vi "Run Test.vi"() -> ()   [LabVIEW 2026, in "Framework Engine.lvclass"]
uses:
  Framework Engine.lvclass
  Framework Engine.lvclass/Framework Engine.ctl
  Domain/Session/Session.lvclass
  Services/Readiness Service/Readines Service.lvclass
  Domain/Test Run Request/Test Run Request.lvclass
  Domain/User/User.lvclass
  Services/Execution Service/Execution Service.lvclass
panel:
  out "error out":errorcluster
  out "Test Run Request":refnum<class "Test Run Request.lvclass">
  in  "Package Version":string
  in  "Package ID":string
  in  "Entry Point":string
  in  "Sequence File Path":path
  in  "Station Name":string
  in  "error in (no error)":errorcluster
  out "Has Permission":bool
  out "Current User":refnum<class "User.lvclass">
  in  "Framework Engine in":refnum<class "Framework Engine.lvclass">
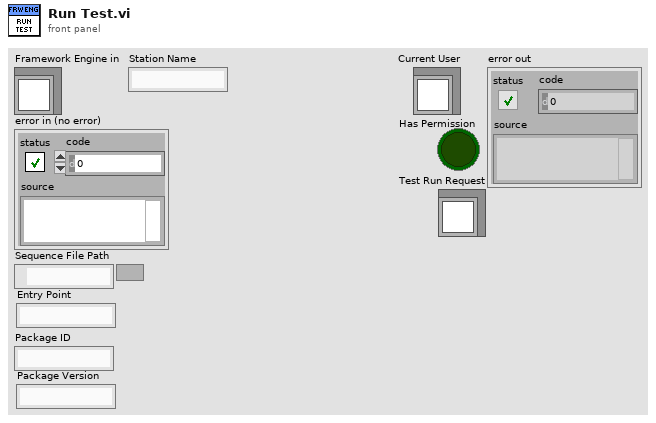
[diagram p1: front panel]
types:
  T1 = typedef "Role Enum.ctl" = enum16{"Operator", "Engineer", "Admin"}
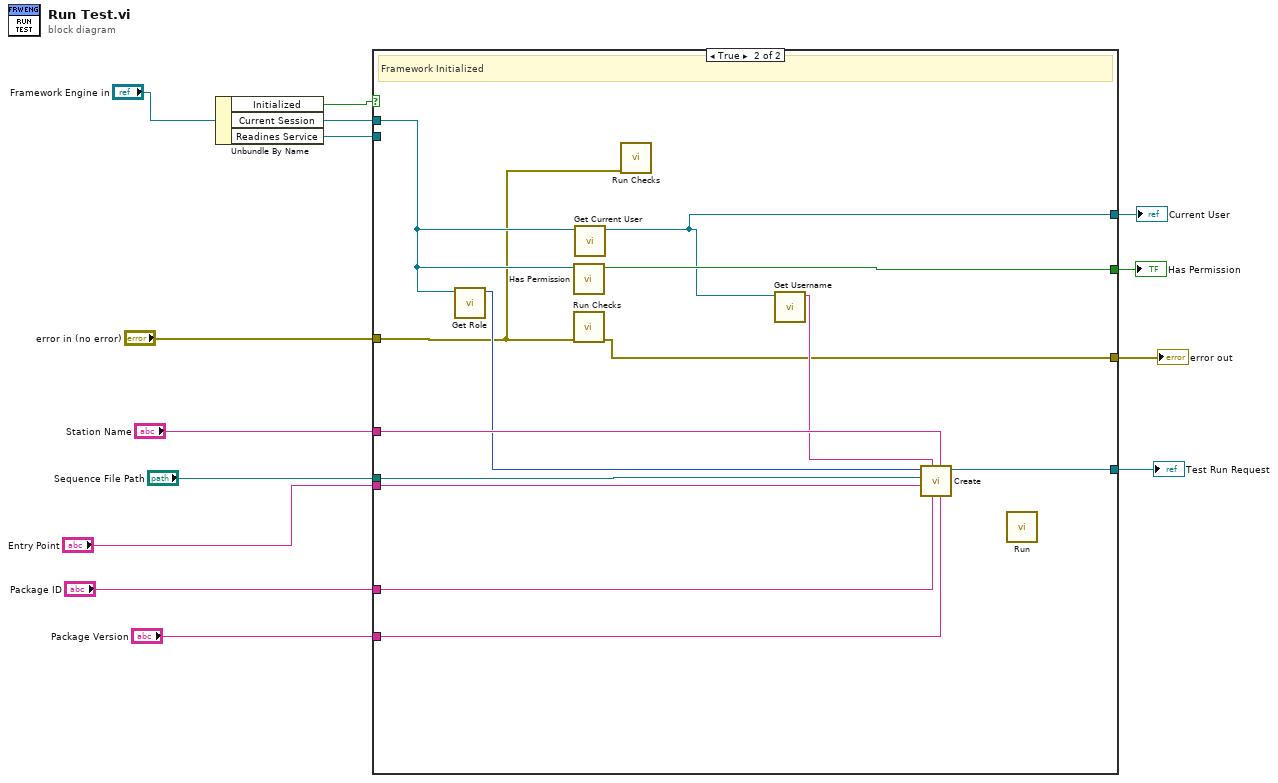
[diagram p0: block diagram]
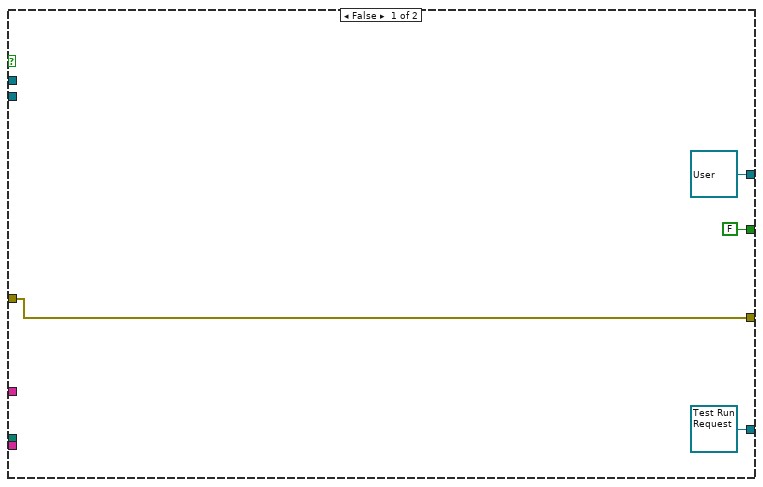
[diagram p2: hidden frame]
diagram:
  n1 = Unbundle By Name("Framework Engine in") -> ("Initialized"=w3:bool, "Current Session"=w10:refnum<class "Session.lvclass">, "Readines Service"=w1:refnum<class "Readines Service.lvclass">)
  n2 = case shown="True" w3 {
    tunnel: [FALSE ("Has Permission") w31] -> w13
    tunnel: "error in (no error)" -> [w18 w19]
    tunnel: "Station Name" -> [_ w30]
    tunnel: w10 -> [_ w29]
    tunnel: [refnum<class "User.lvclass"> refnum ("Current User") w27] -> w9
    tunnel: "Sequence File Path" -> [_ w25]
    tunnel: "Entry Point" -> [_ w24]
    tunnel: "Package ID" -> [_ w23]
    tunnel: "Package Version" -> [_ w22]
    tunnel: [refnum<class "Test Run Request.lvclass"> refnum ("Test Run Request") w21] -> w4
    tunnel: [w18 w20] -> w2
    tunnel: w1 -> [_ _]
    frame False {
    }
    frame True {
      # "Framework Initialized"
      n3 = call "Get Role.vi"("Session Data"=w29) -> ("Role"=w28:T1)  [unwired: 10 in]
      n4 = call "Has Permission.vi"("Session Data"=w29) -> ("Has Permission"=w31:bool)  [unwired: 10 in]
      n5 = call "Run Checks.vi"("error in (no error)"=w19) -> ("error out"=w20:errorcluster)  [unwired: 9 in, 1 out]
      n6 = call "Get Current User.vi"("Session Data"=w29) -> ("Current User"=w27:refnum<class "User.lvclass">)  [unwired: 10 in]
      n7 = call "Run Checks.vi"("error in (no error)"=w19) -> ()  [unwired: 9 in, 2 out]
      n8 = call "Get Username.vi"("User Data"=w27) -> ("Username"=w26:string)  [unwired: 10 in]
      n9 = call "Create.vi"("Package Version"=w22, "Station Name"=w30, "Package ID"=w23, "Current User"=w26, "Entry Point"=w24, "Sequence File Path"=w25, "User Role"=w28) -> ("Test Run Request"=w21:refnum<class "Test Run Request.lvclass">)  [unwired: 4 in]
      n10 = call "Run.vi"() -> ()  [unwired: 12 in]
    }
  }
  "Current User" <- w9
  "Has Permission" <- w13
  "Test Run Request" <- w4
  "error out" <- w2
